vi "String to SubStringInt (SubVI).vi"(10 "Nx4byte":u32, 11 "String in in":string) -> (3 "String out":string)   [LabVIEW 2017, in "LV_Unicorn.lvlib"]
uses:
  LV_Unicorn.lvlib
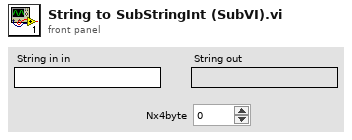
[diagram p1: front panel]
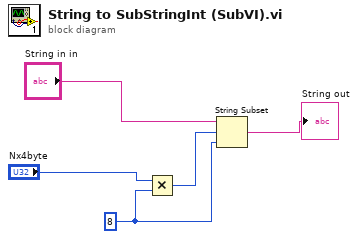
[diagram p0: block diagram]
diagram:
  w3 = u32 8 ("length (rest)")
  n1 = Multiply(x="Nx4byte", y=w3) -> (x*y=w5:u32)
  n2 = String Subset(string="String in in", offset (0)=w5, length (rest)=w3) -> (substring=→"String out":string)
